vi "DFD NStage MRate Filter Design.vi"(4 "filtering mode":T8=2 items=["No Rate Change", "Interpolation", "Decimation"], 5 "manual factorization":i32[](array[numeric]), 6 "fs in [Hz]":dbl=800.0, 7 "factor":i32=8, 8 "error in (no error)":errorcluster, 9 "ripple specs":T1={"passband"=0.1, "stopband"=60.0, "dB/linear? (T: dB)"=TRUE}, 10 "freq specs [Hz]":T7={"fpass"=45.0, "fstop"=52.0}, 11 "using CIC?":bool) -> (0 "error out":errorcluster, 3 "multirate filters out":T2[](array[typedef]) {"mMRate_SumWl" min=1 max=32 step=1; "mMRate_InputIwl" min=1 max=32 step=1; "mMRate_GainWl" min=1 max=32 step=1; "mMRate_OutputWl" min=1 max=32 step=1; "mMRate_InputWl" min=1 max=32 step=1; "mMRate_CoefWl" min=1 max=32 step=1; "mMRate_Mode" items=["Default"=-1, "No Rate Change"=0, "Interpolation"=1, "Decimation"=2, "Interpolated"=3, "Rational"=4]})   [LabVIEW 2017, in "NI_DigFilterLicensed.lvlib"]
doc: "Creates a multistage multirate filter, which meets the requirements you specify by cascading filters in <B>multirate filters out</B>."
uses:
  <vilib>/addons/Digital Filter Design/NI_DigFilterLicensed.lvlib
  <vilib>/addons/Digital Filter Design/_Objects.llb/DFD Multirate Filtering Mode.ctl
  <vilib>/addons/Digital Filter Design/_Objects.llb/DFD Multirate Filter Specification (Design).ctl
  <vilib>/addons/Digital Filter Design/_Objects.llb/DFD Multirate Filter Obj.ctl
  <vilib>/addons/Digital Filter Design/_Objects.llb/DFD Multirate Mode.ctl
  <vilib>/addons/Digital Filter Design/_Objects.llb/DFD Coef Norm Type.ctl
  <vilib>/addons/Digital Filter Design/_Objects.llb/DFD Round-off Mode.ctl
  <vilib>/addons/Digital Filter Design/_Objects.llb/DFD FXP MRate Multiply Mode.ctl
  <vilib>/addons/Digital Filter Design/_Objects.llb/DFD Filter Ripple Specification (Design).ctl
  <vilib>/addons/Digital Filter Design/_Misc.llb/dfd_Error Handlers (Single).vi
  <vilib>/addons/Digital Filter Design/Design.llb/DFD MRate Filter Design (Integer).vi
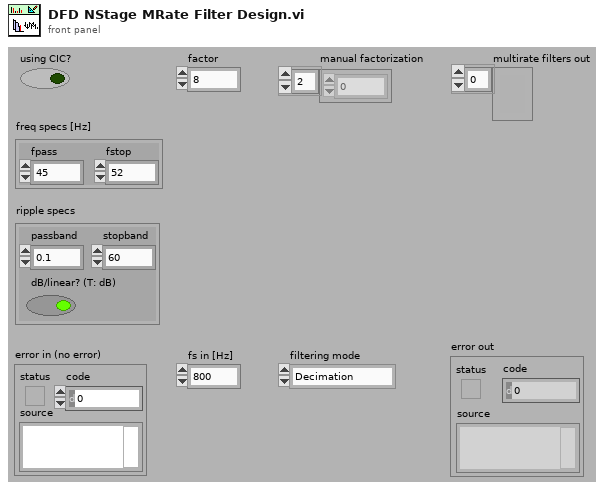
[diagram p1: front panel]
types:
  T1 = typedef "NI_DigFilterLicensed.lvlib/DFD Filter Ripple Specification (Design).ctl" = cluster{"passband":dbl, "stopband":dbl, "dB/linear? (T: dB)":bool}
  T2 = typedef "NI_DigFilterLicensed.lvlib/DFD Multirate Filter Obj.ctl" = cluster{"mMRate_Structure":enum16{"CIC", "FIR", "IIR", "Lattice"}, "mMRate_Mode":T3, "mMRate_Factor":i32, "mMRate_FIRParams":cluster{"mMRate_FIR_H":dbl[], "mMRate_FIR_IsNyquist?":bool, "mMRate_FIR_IsSymmetric?":bool}, "mMRate_CICParams":cluster{"mMRate_CIC_#Stage":i32, "mMRate_CIC_Lag":i32, "mMRate_CIC_Type":enum16{"Lowpass", "Highpass"}}, "mMRate_Order":i32, "mMRate_Version":string, "mMRate_Comments":string, "mMRate_RationalFactor":cluster{"mMRate_L":i32, "mMRate_M":i32}, "mMRate_Fs":dbl, "mMRate_Quantized?":bool, "mMRate_QFilterGain":dbl, "mMRate_CoefWl":i16, "mMRate_Scaling":cluster{"mMRate_ScaleByPowerOf2?":bool, "mMRate_ScaleType":T4}, "mMRate_InputWl":i16, "mMRate_OutputWl":i16, "mMRate_OutputMode":T5, "mMRate_MultMode":T6, "mMRate_BitPruning":bool, "mMRate_GainWl":i16, "mMRate_OutputFwl":i16, "mMRate_SumIwl":i16, "mMRate_InputIwl ":i16, "mMRate_SumWl":i16, "mMRate_CoefIwl":i16}
  T3 = typedef "NI_DigFilterLicensed.lvlib/DFD Multirate Mode.ctl" = i16
  T4 = typedef "NI_DigFilterLicensed.lvlib/DFD Coef Norm Type.ctl" = enum16{"No Norm", "Time Domain 1-Norm", "Time Domain 2-Norm", "Time Domain Inf-Norm"}
  T5 = typedef "NI_DigFilterLicensed.lvlib/DFD Round-off Mode.ctl" = enum16{"Nearest", "Truncation"}
  T6 = typedef "NI_DigFilterLicensed.lvlib/DFD FXP MRate Multiply Mode.ctl" = enum16{"Truncated", "Full"}
  T7 = typedef "NI_DigFilterLicensed.lvlib/DFD Multirate Filter Specification (Design).ctl" = cluster{"fpass":dbl, "fstop":dbl}
  T8 = typedef "NI_DigFilterLicensed.lvlib/DFD Multirate Filtering Mode.ctl" = u16
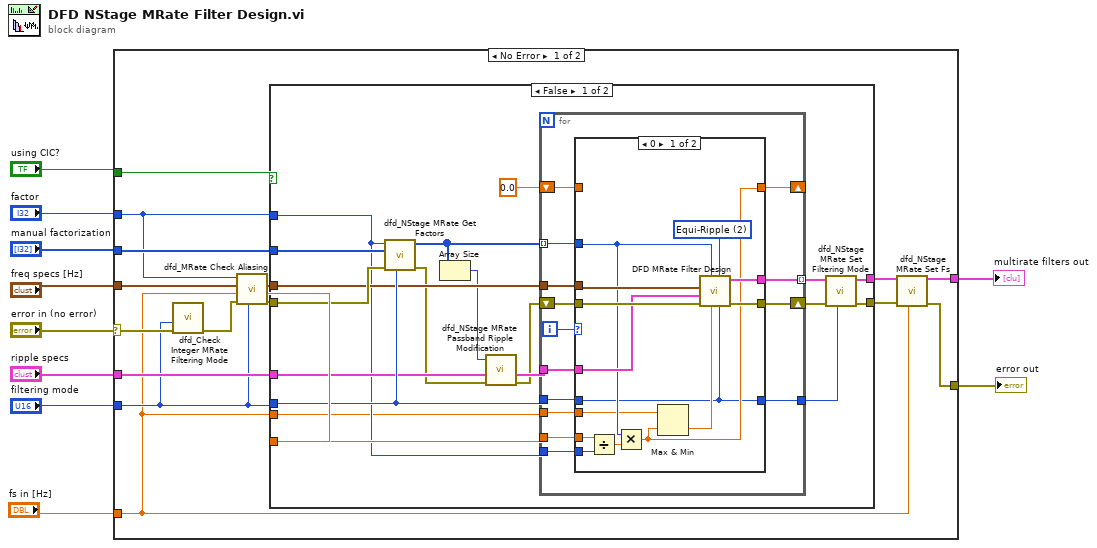
[diagram p0: block diagram]
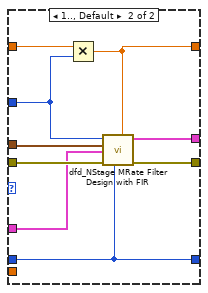
[diagram p2: hidden frame]
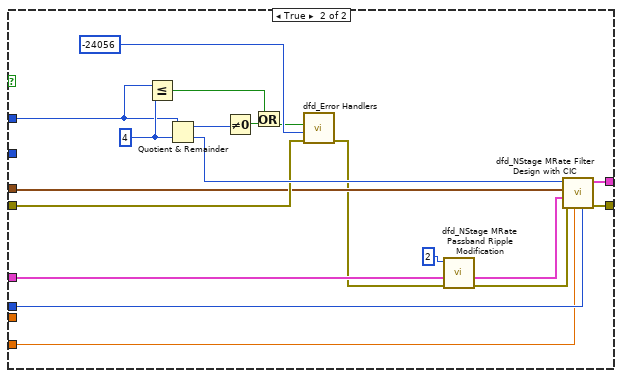
[diagram p3: hidden frame]
diagram:
  n1 = case shown="No Error" "error in (no error)" {
    selector: "error in (no error)" -> [w21 w102]
    tunnel: [w12 w102] -> w3
    tunnel: "using CIC?" -> [w26 _]
    tunnel: "factor" -> [w22 _]
    tunnel: "filtering mode" -> [w15 _]
    tunnel: [w14 _] -> w2
    tunnel: "manual factorization" -> [w24 _]
    tunnel: "freq specs [Hz]" -> [w23 _]
    tunnel: "fs in [Hz]" -> [w11 _]
    tunnel: "ripple specs" -> [w19 _]
    frame No Error {
      n2 = call <vilib>:"dfd_Check Integer MRate Filtering Mode.vi"("error IO"=w21, "filtering mode"=w15) -> ("error out"=w16:errorcluster)  [unwired: 1 in, 8 out]
      n3 = call <vilib>:"dfd_MRate Check Aliasing.vi"("filtering mode"=w15, "error in"=w16, "fs in [Hz]"=w11, "freq specs"=w23, "factor"=w22) -> ("error out"=w17:errorcluster, "filter fs [Hz]"=w18:dbl, "dup freq specs"=w20:T7)  [unwired: 1 in, 3 out]
      n4 = case shown="False" w26 {
        tunnel: w22 -> [w29 w94]
        tunnel: w17 -> [w45 w96]
        tunnel: w15 -> [w39 w90]
        tunnel: [w42 w98] -> w25
        tunnel: [w40 w97] -> w13
        tunnel: w24 -> [w44 _]
        tunnel: w20 -> [w38 w88]
        tunnel: w19 -> [w36 w87]
        tunnel: w18 -> [w30 w89]
        tunnel: w11 -> [w28 _]
        frame False {
          n5 = call <vilib>:"dfd_NStage MRate Get Factors.vi"("filtering mode"=w39, "error in"=w45, "manual factorization"=w44, "factor"=w29) -> ("error out"=w32:errorcluster, "factors"=w35:i32[])  [unwired: 1 in, 5 out]
          n6 = Array Size(array=w35) -> (size(s)=w33:i32)
          n7 = call <vilib>:"dfd_NStage MRate Passband Ripple Modification.vi"("error in (no error)"=w32, "ripple specs"=w36, "#stages"=w33) -> ("error out"=w31:errorcluster, "ripple specs (dB)"=w34:T1)  [unwired: 7 out]
          n8 = for {
            tunnel: w35 -> [w58] mode=indexing
            tunnel: w39 -> [w57]
            tunnel: [w55] -> w43 mode=indexing
            shift-right: [w54] -> w41
            shift-left: w31 -> [w56]
            shift-right: [w53] -> _
            shift-left: 0.0 -> [w52]
            tunnel: [w51] -> w27
            tunnel: w38 -> [w50]
            tunnel: w34 -> [w49]
            tunnel: w30 -> [w48]
            tunnel: w29 -> [w47]
            tunnel: w28 -> [w46]
            i -> [w59]
            n9 = case shown="0" w59 {
              tunnel: w58 -> [w65 w81]
              tunnel: w57 -> [w60 w79]
              tunnel: w56 -> [w73 w80]
              tunnel: [w69 w74] -> w55
              tunnel: [w70 w75] -> w54
              tunnel: [w62 w76] -> w53
              tunnel: w52 -> [_ w82]
              tunnel: [w60 w79] -> w51
              tunnel: w50 -> [w72 w77]
              tunnel: w49 -> [w71 w78]
              tunnel: w48 -> [w67 _]
              tunnel: w47 -> [w66 _]
              tunnel: w46 -> [w63 _]
              frame 0 {
                w64 = u16 2 items=["Kaiser Window", "Dolph-Chebyshev Window", "Equi-Ripple"] ("method")
                n10 = Divide(x=w67, y=w66) -> (x/y=w68:dbl)
                n11 = Multiply(x=w65, y=w68) -> (x*y=w62:dbl)
                n12 = Max & Min(x=w63, y=w62) -> (min(x,y)=w61:dbl)  [unwired: 1 out]
                n13 = call-poly <vilib>:"DFD MRate Filter Design.vi"("filtering mode"=w60, "method"=w64, "fs in [Hz]"=w61, "factor"=w65, "error in (no error)"=w73, "ripple specs"=w71, "freq specs [Hz]"=w72) -> ("error out"=w70:errorcluster, "multirate filter out"=w69:T2)  [unwired: 1 in, 2 out]
              }
              frame 1.., Default {
                n14 = Multiply(x=w82, y=w81) -> (x*y=w76:dbl)
                n15 = call <vilib>:"dfd_NStage MRate Filter Design with FIR.vi"("fs [Hz]"=w76, "filtering mode"=w79, "error in"=w80, "ripple specs"=w78, "freq spec"=w77, "current factor"=w81) -> ("error out"=w75:errorcluster, "multirate filter out"=w74:T2)  [unwired: 2 in, 2 out]
              }
            }
          }
          n16 = call <vilib>:"dfd_NStage MRate Set Filtering Mode.vi"("filtering mode"=w27, "error in (no error)"=w41, "multirate filter in"=w43) -> ("error out"=w40:errorcluster, "multirate filter out"=w42:T2[])  [unwired: 7 out]
        }
        frame True {
          w95 = 4 ("y")
          n17 = Less Or Equal?(x=w94, y=w95) -> (x <= y?=w92:bool)
          n18 = Quotient & Remainder(x=w94, y=w95) -> (x-y*floor(x/y)=w101:i32, floor(x/y)=w99:i32)
          n19 = Not Equal To 0?(x=w101) -> (x != 0?=w91:bool)
          n20 = Or(x=w92, y=w91) -> (x .or. y?=w93:bool)
          n21 = call-poly <vilib>:"dfd_Error Handlers.vi"("error in (no error)"=w96, "error code"=-24056 ("ERR_FACOTR_CANNOT_DIVIDE"), "condition failed?"=w93) -> ("error out"=w84:errorcluster)  [unwired: 8 out]
          n22 = call <vilib>:"dfd_NStage MRate Passband Ripple Modification.vi"("error in (no error)"=w84, "ripple specs"=w87, "#stages"=2) -> ("error out"=w83:errorcluster, "ripple specs (dB)"=w86:T1)  [unwired: 7 out]
          n23 = call <vilib>:"dfd_NStage MRate Filter Design with CIC.vi"("filtering mode"=w90, "fs [Hz]"=w89, "error in (no error)"=w83, "ripple specs"=w86, "freq spec"=w88, "CIC factor"=w99) -> ("error out"=w97:errorcluster, "multirate filters out"=w98:T2[])  [unwired: 4 out]
        }
      }
      n24 = call <vilib>:"dfd_NStage MRate Set Fs.vi"("fs in [Hz]"=w11, "error in (no error)"=w13, "multirate filter in"=w25) -> ("error out"=w12:errorcluster, "multirate filter out"=w14:T2[])  [unwired: 7 out]
    }
    frame Error {
    }
  }
  "error out" <- w3
  "multirate filters out" <- w2
